vi "CRCCalculate_CRC校验计算.vi"(1 "原始指令":string) -> (0 "带CRC校验指令":string)   [LabVIEW 2011]
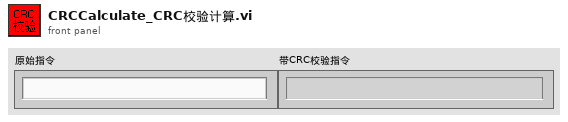
[diagram p1: front panel]
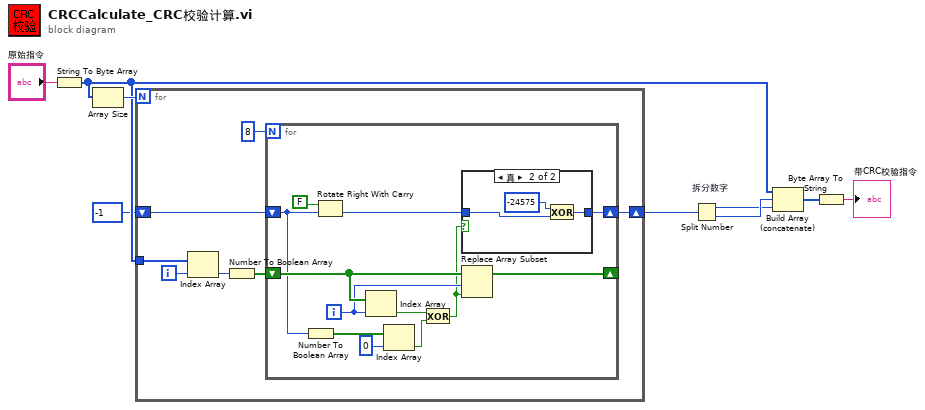
[diagram p0: block diagram]
diagram:
  n1 = String To Byte Array(string="原始指令") -> (unsigned byte array=w3:u8[])
  n2 = Array Size(array=w3) -> (size(s)=w9:i32)
  n3 = for {
    N: w9 -> [_]
    shift-right: [w13] -> w1
    shift-left: i16 -1 -> [w12]
    tunnel: w3 -> [w10]
    i -> [w16]
    n4 = Index Array(array=w10, index=w16) -> (element=w15:u8)
    n5 = Number To Boolean Array(number=w15) -> (Boolean array=w14:bool[])
    n6 = for {
      N: 8 -> [_]
      shift-right: [w23] -> _
      shift-left: w14 -> [w28]
      shift-right: [w17] -> w13
      shift-left: w12 -> [w18]
      i -> [w22]
      n7 = Number To Boolean Array(number=w18) -> (Boolean array=w27:bool[])
      n8 = Rotate Right With Carry(2:w18, 3:FALSE ("进位")) -> (0:w19:i16)  [unwired: 1 out]
      n9 = Index Array(array=w28, index=w22) -> (element=w25:bool)
      n10 = Index Array(array=w27, index=0 ("索引")) -> (element=w24:bool)
      n11 = Exclusive Or(1:w24, 2:w25) -> (0:w20:bool)
      n12 = case shown="真" w20 {
        tunnel: w19 -> [w29 w32]
        tunnel: [w29 w30] -> w17
        frame False {
        }
        frame True {
          n13 = Exclusive Or(1:w32, 2:i16 -24575 ("x")) -> (0:w30:i16)
        }
      }
      n14 = Replace Array Subset(array=w28, new element=w20, index=w22) -> (w23:bool[])
    }
  }
  n15 = Split Number "拆分数字"(x=w1) -> (hi(x)=w6:u8, lo(x)=w7:u8)
  n16 = Build Array (concatenate)(w3, w7, w6) -> (w5:u8[])
  n17 = Byte Array To String(unsigned byte array=w5) -> (string=→"带CRC校验指令":string)
